vi "2016RefLoopPulseGen_Original.vi"() -> ()   [LabVIEW 2015]
uses:
  <vilib>/express/express arith-compare/Formula/XNode/ExpressFormulaBlockNode.xnode
  <vilib>/express/express shared/transition.llb/Dynamic To Waveform Array.vi
  <vilib>/express/express arith-compare/Formula/Block/exnFormulaBlock how many pts in the wave.vi
  <vilib>/express/express shared/ex_Modify Signal Name.vi
  <vilib>/express/express shared/transition.llb/Waveform Array To Dynamic.vi
  <vilib>/addons/control/pid/NI_PID_autopid.lvlib
  <vilib>/DAQmx/write.llb/DAQmx Write (Digital 1D Bool 1Chan 1Samp).vi
  <vilib>/Utility/error.llb/DialogType.ctl
  <vilib>/express/express signal manip/GetorSetDDTAttributes/Set DDT Attributes/Set DDT Properties.xnode
  <vilib>/express/express signal manip/GetorSetDDTAttributes/Set DDT Attributes/SetT0.vi
  <vilib>/DAQmx/configure/timing.llb/DAQmx Timing (Sample Clock).vi
  <vilib>/DAQmx/configure/timing.llb/DAQmx Timing (Implicit).vi
  <vilib>/DAQmx/create/channels.llb/DAQmx Create Channel (CO-Pulse Generation-Frequency).vi
  <vilib>/DAQmx/write.llb/DAQmx Write (Digital 1D Bool NChan 1Samp 1Line).vi
  <vilib>/DAQmx/read.llb/DAQmx Read (Analog 1D DBL NChan 1Samp).vi
panel:
  out "Loop Time":dbl
  in  "stop 4":bool
  in  "?":bool
  out "error out 2":errorcluster
  out "error out":errorcluster
  in  "output duty cycle range 1":cluster{"output high":dbl, "output low":dbl}={"output high"=100.0, "output low"=0.0}
  out "Waveform Chart":dbl(graph)=1.0280585289001465
  out "Elapsed Time (s)":dbl=1192.0481810569763
  in  "?":T1(tab)
  in  "Lower Test Section offset":dbl
  in  "Separator T offset":dbl
  in  "Liquid Tank P offset":dbl=8500.0
  out "Test Section P (Pa)":dbl=116198.57530062649
  in  "P atm":dbl=101325.0
  in  "Liquid Inlet Offset":dbl=1100.0
  in  "Upper Test Sec":dbl
  in  "Dev Section P offset":dbl=-15000.0
  in  "Liquid Inlet T offset":dbl
  in  "Vapor Inlet T offset":dbl
  in  "Liquid Tank T offset":dbl
  in  "Vapor Tank T offset":dbl
  in  "Separator P Offset":dbl=2500.0
  out "Liquid Tank Heater Temp. [C]":dbl=-0.00013997779130803294 format="%#_4g"
  out "Vapor Tank Heater Temp. [C]":dbl=-0.00010921620483495026 format="%#_4g"
  in  "Vapor Tank Heater [V]":dbl(slide) scale=0.0..10.0
  in  "Liquid Tank Heater [V]":dbl(slide) scale=0.0..10.0
  out "Quality\n[-]":dbl=0.5124735258578829 format="%#_3f"
  out "Mixture Enthalpy":dbl=315341.8738601937
  out "Upper TS Sat. Temp. [C]":dbl=-30.741985921320232 format="%#_4g"
  out "Upper Test Section 2\n(not connected)":dbl=19080.10707676887
  out "?":dbl=nan format="%#_4g"
  out "?":dbl=nan format="%#_4g"
  out "Vapor Inlet Sat. Temp. [C]":dbl=18.983650599672455 format="%#_4g"
  out "Liquid Inlet Sat. Temp. [C]":dbl=18.967113726868046 format="%#_4g"
  out "Separator Sat. Temp. [C]":dbl=18.962084458713754 format="%#_4g"
  out "Liquid Tank Sat. Temp. [C]":dbl=17.336038014955804 format="%#_4g"
  out "Vapor Tank Sat. Temp. [C]":dbl=nan format="%#_4g"
  out "Lower Test Section 2\n(not connected)":dbl=-5.945274707393333 format="%#_6f"
  out "Streamwise":dbl=-4309.180034596612 format="%#_2e"
  out "Dev Section":dbl=117529.39865406745 format="%#_5f"
  out "Separator 2":dbl=117436.76445279745 format="%#_5f"
  out "Vapor Tank 2\n(need replaced)":dbl=-34009.73110511369 format="%#_6f"
  out "Liquid Inlet 2":dbl=117458.36040777806 format="%#_5f"
  out "Liquid Tank 2":dbl=119158.55398835387 format="%#_5f"
  out "Upper TS Sat. Pres.":dbl=117745.79282373996
  out "Upper Test Section":dbl=19.02953821278611 format="%#_4g"
  out "Lower Test Section":dbl=18.841711969674257 format="%#_4g"
  out "Vapor Inlet":dbl=19.940090617924646 format="%#_4g"
  out "Liquid Inlet":dbl=19.29273815741822 format="%#_4g"
  out "Separator":dbl=19.351746784304748 format="%#_4g"
  out "Liquid Tank":dbl=19.064732737324512 format="%#_4g"
  out "Vapor Tank":dbl=19.311251471245498 format="%#_4g"
  out "Liquid Inlet Sat. Pres.":dbl=118921.18754866866 format="%#_4f"
  out "Liquid Tank Sat. Pres.":dbl=117902.28866165497 format="%#_4f"
  out "Vapor Inlet Sat. Pres.":dbl=119186.31350697557 format="%#_4f"
  out "Lower Test Section Sat. Pres.":dbl=116914.11104502712 format="%#_4f"
  out "Separator Sat. Pres.":dbl=121862.28710047182 format="%#_4f"
  out "Vapor Tank Sat. Pres.":dbl=119004.3043776936 format="%#_4f"
  out "Evaporator Bottom":dbl=0.07812510710210246 format="%#_4g"
  out "Evaporator Top":dbl=-55440.10937765434 format="%#_4g"
  out "Condenser Bottom":dbl=-0.00013633631982423782 format="%#_4g"
  out "Condenser Top":dbl=-0.0001304783004807413 format="%#_4g"
  in  "Save File":bool
  out "StaticPressDiff(Pa)":dbl=-222.00009683752145
  out "DC":dbl
  out "Numeric":dbl=2.098083621149279e-08
  out "Pressure Drop":dbl=2.6226045264365988e-08
  in  "Boolean 2":bool
  out "Camera Voltage":dynamicdata(graph)
  in  "Pitot Offset [Pa]":dbl
  in  "PG-TS Offset\n[Pa]":dbl
  in  "Send Pulse 2":bool
  out "Psat liq":dbl=119.96937909943745
  in  "Save Loop Data":bool
  in  "Boolean":bool
  in  "Sampling frequency (Hz)":dbl=1000.0
  in  "Length of recording (s)":dbl=2.0
  in  "PG Abs Offset":dbl=11500.0
  out "Psat vap":dbl=121.24568157832624
  out "Pitot Amps":dbl=2.6415199999999147e-07
  out "dP Pitot Probe":dynamicdata(graph)=[{"t0"=timestamp(3554308544.5452676 s since 1904-01-01), "dt"=0.001, "Y"=array[2000 elements], "attributes"=variant("NI_ChannelName"=variant(string "Pitot dP (Formula Result)"), "NI_OriginalChannelName"=variant(string "Pitot dP"), "NI_UnitDescription"=variant(string "Amps"))}]
  out "Tank Pressure":dynamicdata(graph)=[{"t0"=timestamp(3554308544.5452676 s since 1904-01-01), "dt"=0.001, "Y"=array[2000 elements], "attributes"=variant("NI_ChannelName"=variant(string "Abs P (Formula Result)"), "NI_OriginalChannelName"=variant(string "Abs P"), "NI_UnitDescription"=variant(string "Volts"))}]
  out "dP to test section":dynamicdata(graph)=[{"t0"=timestamp(3554308544.5452814 s since 1904-01-01), "dt"=0.001, "Y"=array[2000 elements], "attributes"=variant("NI_ChannelName"=variant(string "PG to TS dP (Formula Result)"), "NI_OriginalChannelName"=variant(string "PG to TS dP"), "NI_UnitDescription"=variant(string "Volts"))}]
  out "Pitot dP":dbl=-4308.9404273994505
  out "Liquid Temp":dbl=19.52526901660894
  out "Vapor Temp":dbl=19.805676371442082
  in  "CCW":bool
  in  "?":bool
  out "Loop iterations":i32
  in  "Send Pulse":bool
  in  "Steps":i32=10000 min=0 max=40000 step=500
  in  "Idle State":i32(ring)=10214 items=["High"=10192, "Low"=10214]
  in  "Counter(s)":tag="cDAQ1Mod8/ctr0" caption="Counter"
  in  "Duty Cycle":dbl=0.5 min=0.1 max=1.0 step=0.1
  in  "Frequency (Hz)":dbl=1000.0 min=0.0 max=10000.0 step=500.0
  out "Mass Flow Rate":dbl=nan
  in  "Heaters":bool
  out "PG Abs":dbl=119484.80284900061
  out "PG to TS dP":dbl=4351.8068090218785
  in  "Save dP data":bool
  out "dP [Pa]  W1 to W7":dbl=-0.008208439355650089
  out "dP [Pa] W1 to W4":dbl=0.008075495341450085
  in  "stop":bool
  in  "reinitialize? (F) 2":bool=TRUE
  out "Liquid Mass Flow Rate":cluster{"[0]":dbl, "[1]":dbl}(graph)={"[0]"=0.0, "[1]"=-94.2977673785965}
  out "Voltage Out 2":dbl
  out "Liquid Line Density [g/cm3]":dbl=-0.5000013113022632
  out "Liquid Flow Rate [g/s]":dbl=-94.2977673785965
  in  "LiquidOnOff":bool
  in  "LiquidManPID":bool
  in  "PID gains 2":T2={"proportional gain (Kc)"=1e-15, "integral time (Ti, min)"=1e-12, "derivative time (Td, min)"=1e-12} {"derivative time (Td, min)" format="%.4e"; "integral time (Ti, min)" format="%.4e"; "proportional gain (Kc)" format="%.4e"}
  in  "output range 2":cluster{"output high":dbl, "output low":dbl}={"output high"=4.5, "output low"=2.0} {"output low" format="%.2f"; "output high" format="%.2f"}
  in  "Valve Voltage [V] 2":dbl=2.6 format="%.2f"
  in  "Liquid Flow Set Point\n[g/s]":dbl format="%.2f"
  in  "output range":cluster{"output high":dbl, "output low":dbl}={"output high"=3.0, "output low"=2.0} {"output low" format="%.2f"; "output high" format="%.2f"}
  in  "PID gains":T2={"proportional gain (Kc)"=1e-14, "integral time (Ti, min)"=1e-12, "derivative time (Td, min)"=1e-12} {"derivative time (Td, min)" format="%.4e"; "integral time (Ti, min)" format="%.4e"; "proportional gain (Kc)" format="%.4e"}
  in  "VaporManPID":bool
  in  "VaporOnOff":bool
  in  "Vapor Flow Set Point\n[g/s]":dbl format="%.2f"
  in  "Valve Voltage [V]":dbl=2.33 format="%.2f"
  out "Vapor Line Density [g/cm3]":dbl=-0.5000029504300922
  out "Vapor Flow Rate [g/s]":dbl=-94.29782933653023
  out "Voltage Out":dbl
  out "Vapor Mass Flow Rate":cluster{"[0]":dbl, "[1]":dbl}(graph)
  in  "reinitialize? (F)":bool=TRUE
  in  "PID on 2":bool
  in  "T1 Setpoint [C]":dbl format="%.2f"
  in  "reinitialize? (F) 3":bool=TRUE
  in  "PID gains 3":T2={"proportional gain (Kc)"=1e-14, "integral time (Ti, min)"=1e-12, "derivative time (Td, min)"=1e-12} {"derivative time (Td, min)" format="%.4e"; "integral time (Ti, min)" format="%.4e"; "proportional gain (Kc)" format="%.4e"}
  out "T1":cluster{"[0]":dbl, "[1]":dbl}(graph)
  out "T1 Measured [C]":dbl
  out "DutyCycleCalc1":dbl format="%.6f"
  in  "T2 Setpoint [C]":dbl format="%.2f"
  in  "reinitialize? (F) 4":bool=TRUE
  in  "PID gains 4":T2={"proportional gain (Kc)"=1e-14, "integral time (Ti, min)"=1e-12, "derivative time (Td, min)"=1e-12} {"derivative time (Td, min)" format="%.4e"; "integral time (Ti, min)" format="%.4e"; "proportional gain (Kc)" format="%.4e"}
  out "T2":cluster{"[0]":dbl, "[1]":dbl}(graph)
  out "T2 Measured [C]":dbl
  out "DutyCycleCalc2":dbl format="%.6f"
  in  "stop 2":bool
  in  "PID on":bool
  in  "PID on 3":bool
  in  "T3 Setpoint [C]":dbl format="%.2f"
  in  "reinitialize? (F) 5":bool=TRUE
  in  "PID gains 5":T2={"proportional gain (Kc)"=1e-14, "integral time (Ti, min)"=1e-12, "derivative time (Td, min)"=1e-12} {"derivative time (Td, min)" format="%.4e"; "integral time (Ti, min)" format="%.4e"; "proportional gain (Kc)" format="%.4e"}
  out "T3":cluster{"[0]":dbl, "[1]":dbl}(graph)
  out "T3 Measured [C]":dbl
  out "DutyCycleCalc3":dbl format="%.6f"
  in  "PID on 4":bool
  in  "T4 Setpoint [C]":dbl format="%.2f"
  in  "reinitialize? (F) 6":bool=TRUE
  in  "PID gains 6":T2={"proportional gain (Kc)"=1e-14, "integral time (Ti, min)"=1e-12, "derivative time (Td, min)"=1e-12} {"derivative time (Td, min)" format="%.4e"; "integral time (Ti, min)" format="%.4e"; "proportional gain (Kc)" format="%.4e"}
  out "T4":cluster{"[0]":dbl, "[1]":dbl}(graph)
  out "T4 Measured [C]":dbl
  out "DutyCycleCalc4":dbl format="%.6f"
  in  "PID on 5":bool
  in  "T5 Setpoint [C]":dbl format="%.2f"
  in  "reinitialize? (F) 7":bool=TRUE
  in  "PID gains 7":T2={"proportional gain (Kc)"=1e-14, "integral time (Ti, min)"=1e-12, "derivative time (Td, min)"=1e-12} {"derivative time (Td, min)" format="%.4e"; "integral time (Ti, min)" format="%.4e"; "proportional gain (Kc)" format="%.4e"}
  out "T5":cluster{"[0]":dbl, "[1]":dbl}(graph)
  out "T5 Measured [C]":dbl
  out "DutyCycleCalc5":dbl format="%.6f"
  in  "PID on 6":bool
  in  "T6 Setpoint [C]":dbl format="%.2f"
  in  "reinitialize? (F) 8":bool=TRUE
  in  "PID gains 8":T2={"proportional gain (Kc)"=1e-14, "integral time (Ti, min)"=1e-12, "derivative time (Td, min)"=1e-12} {"derivative time (Td, min)" format="%.4e"; "integral time (Ti, min)" format="%.4e"; "proportional gain (Kc)" format="%.4e"}
  out "T6":cluster{"[0]":dbl, "[1]":dbl}(graph)
  out "T6 Measured [C]":dbl
  out "DutyCycleCalc6":dbl format="%.6f"
  in  "PID on 7":bool
  in  "T7 Setpoint [C]":dbl format="%.2f"
  in  "reinitialize? (F) 9":bool=TRUE
  in  "PID gains 9":T2={"proportional gain (Kc)"=1e-14, "integral time (Ti, min)"=1e-12, "derivative time (Td, min)"=1e-12} {"derivative time (Td, min)" format="%.4e"; "integral time (Ti, min)" format="%.4e"; "proportional gain (Kc)" format="%.4e"}
  out "T7":cluster{"[0]":dbl, "[1]":dbl}(graph)
  out "T7 Measured [C]":dbl
  out "DutyCycleCalc7":dbl format="%.6f"
  out "WinOn 2":bool
  out "WinOn 1":bool
  in  "PID on 8":bool
  in  "T8 Setpoint [C]":dbl format="%.2f"
  in  "reinitialize? (F) 10":bool=TRUE
  in  "PID gains 10":T2={"proportional gain (Kc)"=1e-14, "integral time (Ti, min)"=1e-12, "derivative time (Td, min)"=1e-12} {"derivative time (Td, min)" format="%.4e"; "integral time (Ti, min)" format="%.4e"; "proportional gain (Kc)" format="%.4e"}
  out "T8":cluster{"[0]":dbl, "[1]":dbl}(graph)
  out "T8 Measured [C]":dbl
  out "DutyCycleCalc8":dbl format="%.6f"
  in  "PID on 9":bool
  in  "T9 Setpoint [C]":dbl format="%.2f"
  in  "reinitialize? (F) 11":bool=TRUE
  in  "PID gains 11":T2={"proportional gain (Kc)"=1e-14, "integral time (Ti, min)"=1e-12, "derivative time (Td, min)"=1e-12} {"derivative time (Td, min)" format="%.4e"; "integral time (Ti, min)" format="%.4e"; "proportional gain (Kc)" format="%.4e"}
  out "T9":cluster{"[0]":dbl, "[1]":dbl}(graph)
  out "T9 Measured [C]":dbl
  out "DutyCycleCalc9":dbl format="%.6f"
  in  "PID on 10":bool
  in  "T10 Setpoint [C]":dbl format="%.2f"
  in  "reinitialize? (F) 12":bool=TRUE
  in  "PID gains 12":T2={"proportional gain (Kc)"=1e-14, "integral time (Ti, min)"=1e-12, "derivative time (Td, min)"=1e-12} {"derivative time (Td, min)" format="%.4e"; "integral time (Ti, min)" format="%.4e"; "proportional gain (Kc)" format="%.4e"}
  out "T10":cluster{"[0]":dbl, "[1]":dbl}(graph)
  out "T10 Measured [C]":dbl
  out "DutyCycleCalc10":dbl format="%.6f"
  in  "PID on 11":bool
  in  "T11 Setpoint [C]":dbl format="%.2f"
  in  "reinitialize? (F) 13":bool=TRUE
  in  "PID gains 13":T2={"proportional gain (Kc)"=1e-14, "integral time (Ti, min)"=1e-12, "derivative time (Td, min)"=1e-12} {"derivative time (Td, min)" format="%.4e"; "integral time (Ti, min)" format="%.4e"; "proportional gain (Kc)" format="%.4e"}
  out "T11":cluster{"[0]":dbl, "[1]":dbl}(graph)
  out "T11 Measured [C]":dbl
  out "DutyCycleCalc11":dbl format="%.6f"
  in  "PID on 12":bool
  in  "T12 Setpoint [C]":dbl format="%.2f"
  in  "reinitialize? (F) 14":bool=TRUE
  in  "PID gains 14":T2={"proportional gain (Kc)"=1e-14, "integral time (Ti, min)"=1e-12, "derivative time (Td, min)"=1e-12} {"derivative time (Td, min)" format="%.4e"; "integral time (Ti, min)" format="%.4e"; "proportional gain (Kc)" format="%.4e"}
  out "T12":cluster{"[0]":dbl, "[1]":dbl}(graph)
  out "T12 Measured [C]":dbl
  out "DutyCycleCalc12":dbl format="%.6f"
  in  "PID on 13":bool
  in  "T13 Setpoint [C]":dbl format="%.2f"
  in  "reinitialize? (F) 15":bool=TRUE
  in  "PID gains 15":T2={"proportional gain (Kc)"=1e-14, "integral time (Ti, min)"=1e-12, "derivative time (Td, min)"=1e-12} {"derivative time (Td, min)" format="%.4e"; "integral time (Ti, min)" format="%.4e"; "proportional gain (Kc)" format="%.4e"}
  out "T13":cluster{"[0]":dbl, "[1]":dbl}(graph)
  out "T13 Measured [C]":dbl
  out "DutyCycleCalc13":dbl format="%.6f"
  in  "PID on 14":bool
  in  "T14 Setpoint [C]":dbl format="%.2f"
  in  "reinitialize? (F) 16":bool=TRUE
  in  "PID gains 16":T2={"proportional gain (Kc)"=1e-14, "integral time (Ti, min)"=1e-12, "derivative time (Td, min)"=1e-12} {"derivative time (Td, min)" format="%.4e"; "integral time (Ti, min)" format="%.4e"; "proportional gain (Kc)" format="%.4e"}
  out "T14":cluster{"[0]":dbl, "[1]":dbl}(graph)
  out "T14 Measured [C]":dbl
  out "DutyCycleCalc14":dbl format="%.6f"
  # "Same button as Save data loop button on Pulse Generator tab"
  # "Test Section Properties"
  # "Pressure\n[Pa]"
  # "Sat. Temp.\n[C]"
  # "Sat. Pressure\n[Pa]"
  # "Temp.\n[C]"
  # "Temperature [C]"
  # "Condenser"
  # "Evaporator"
  # "Top"
  # "Bottom"
  # "Save File"
  # "Do Not\nSave File"
  # "In order to send a  group of pulses follow the steps below.\n1)Press the button labeled Send Pulse\n2)Press the button a second time in order to prepare for another pulse\n3)Press the stop button to reset the Send Pulse button\n4)Repeat process for next pulse\n\nNote: 1000 steps is a full cycle of the valve, this will send one pulse"
  # "Saving Data:\n\n- Press the Save Loop Data button to record time-averaged (every 2s) data from the loop (data from Test Section Properties tab). Pressing the button again keeps writing in the same file.\n\n-Press the Save dP data to record time resolved data. Each time you press the button, a new file is recorded."
  # "Pulse Generator\nTemperatures"
  # "Vapor Side"
  # "Valve On"
  # "Valve Off"
  # "Manual Flow\nControl"
  # "PID Flow\nControl"
  # "Liquid Side"
  # "Valve On"
  # "Valve Off"
  # "Manual Flow\nControl"
  # "PID Flow\nControl"
  # "Heater On"
  # "Heater On"
  # "Heater On"
  # "Heater On"
  # "Heater Off"
  # "Heater Off"
  # "Heater Off"
  # "Heater Off"
  # "Heater On"
  # "Heater On"
  # "Heater On"
  # "Heater Off"
  # "Heater Off"
  # "Heater Off"
  # "Heater On"
  # "Heater On"
  # "Heater On"
  # "Heater On"
  # "Heater Off"
  # "Heater Off"
  # "Heater Off"
  # "Heater Off"
  # "Heater On"
  # "Heater On"
  # "Heater On"
  # "Heater Off"
  # "Heater Off"
  # "Heater Off"
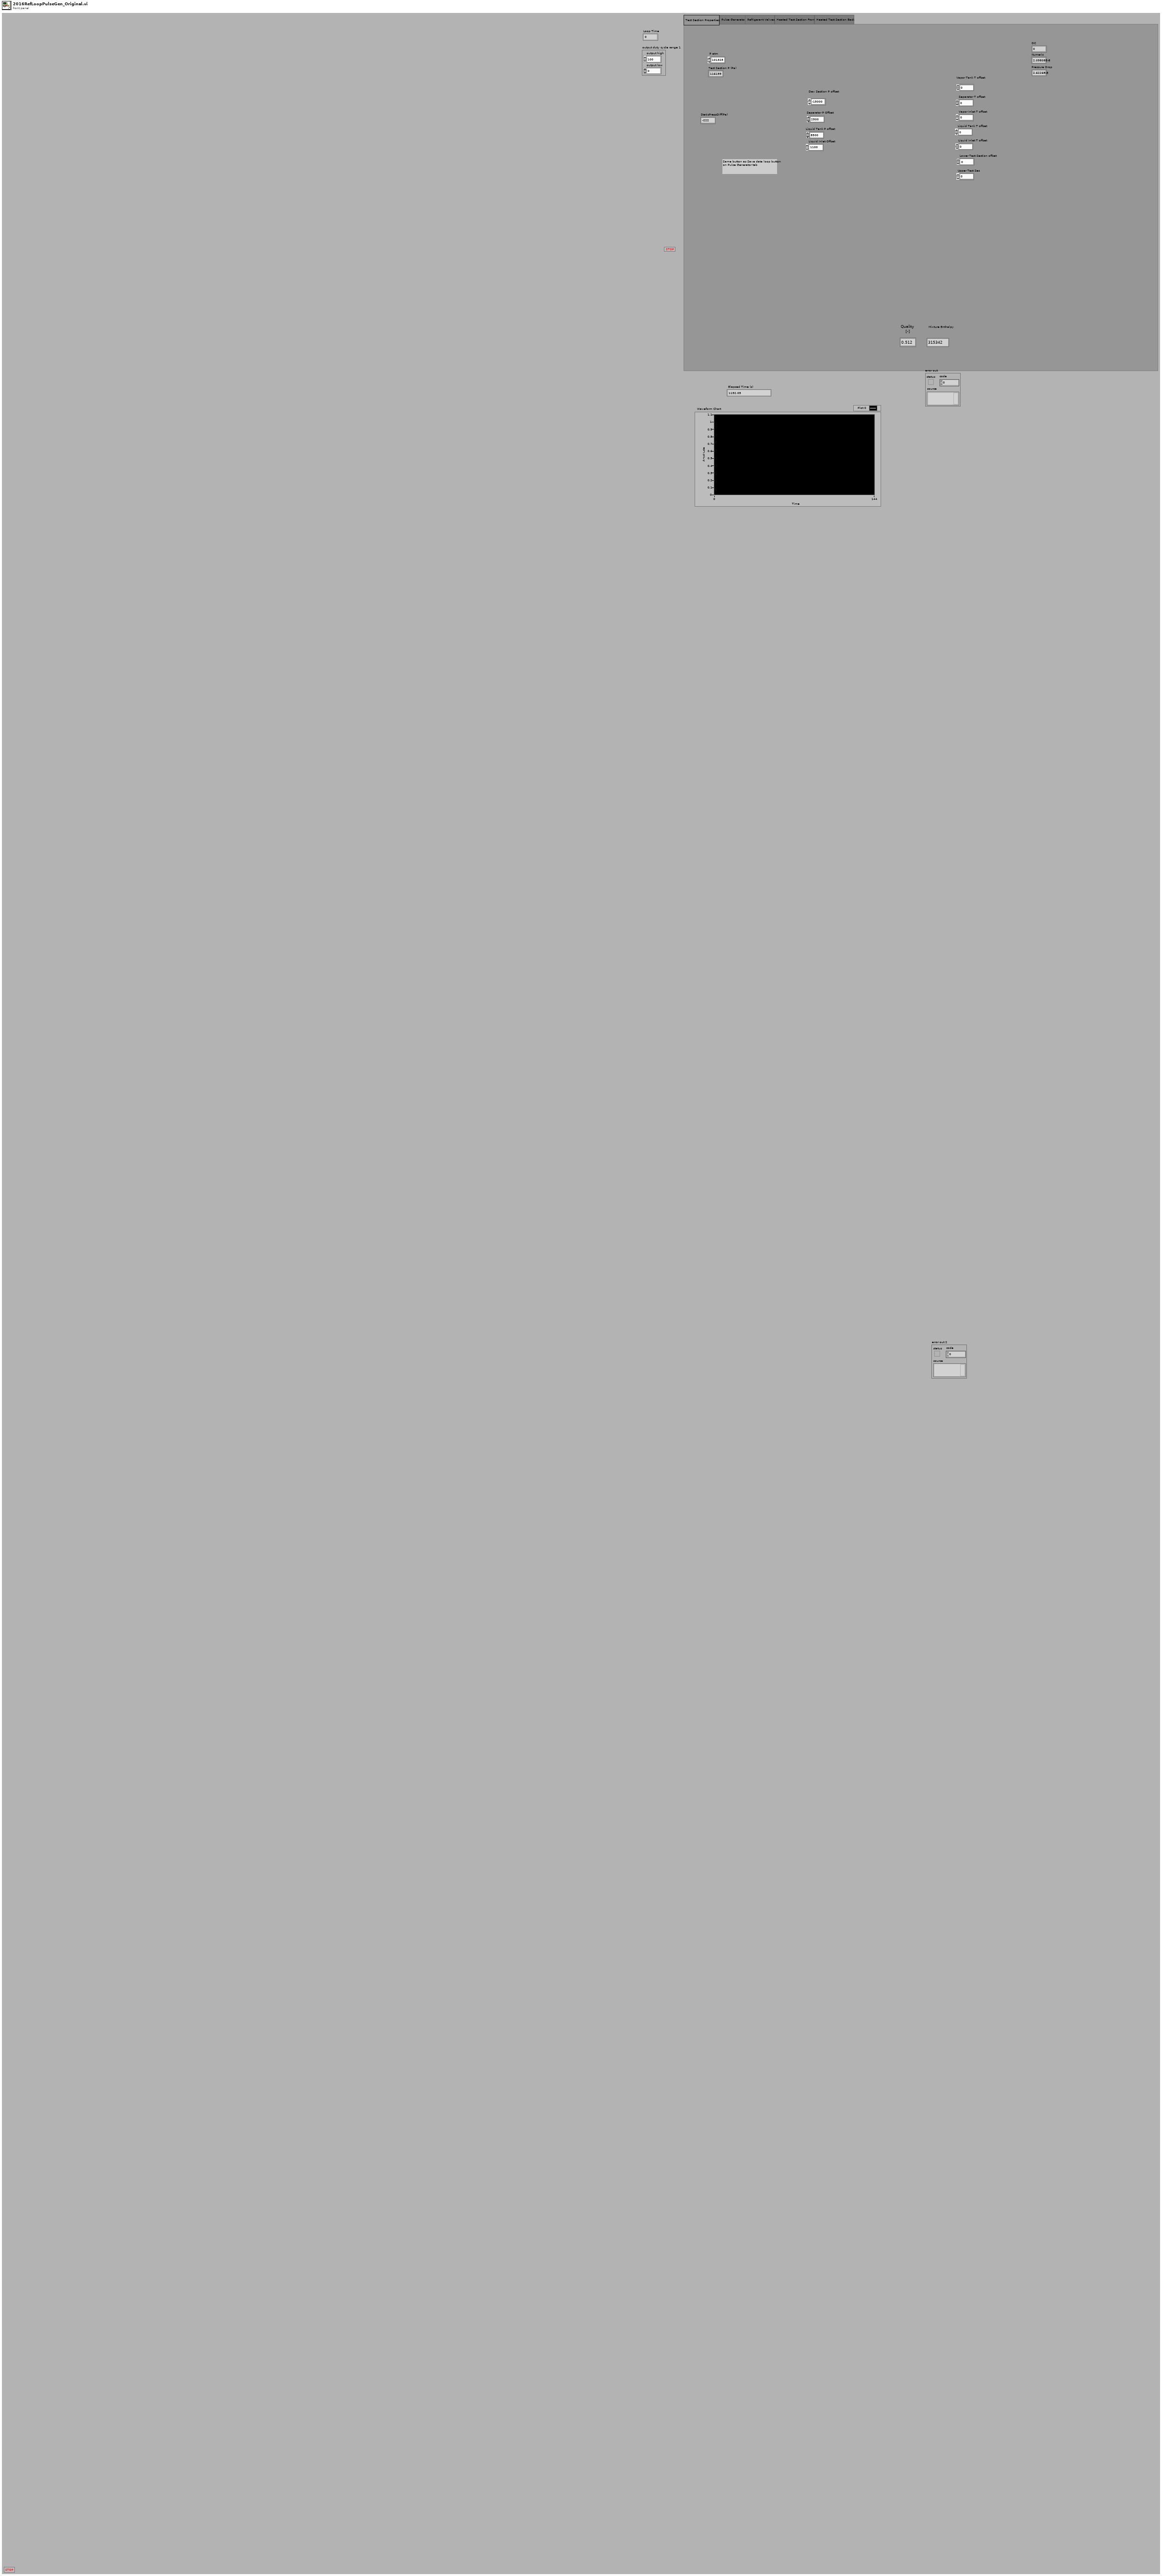
[diagram p1: front panel]
types:
  T1 = enum32{"Test Section Properties", "Pulse Generator", "Refrigerant Valves", "Heated Test Section Front", "Heated Test Section Back"}
  T2 = cluster{"proportional gain (Kc)":dbl, "integral time (Ti, min)":dbl, "derivative time (Td, min)":dbl}
  T3 = typedef "DialogType.ctl" = u16
  T4 = cluster{bool[], bool[], bool[], bool[], bool[], bool[], bool[], bool[], bool[], bool[], bool[], bool[], bool[], bool[]}
  T5 = cluster{"controller type":u16, "relay cycles":i32, "relay amplitude":dbl, "control specification":u16, "PV noise level":dbl}
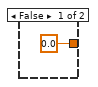
[diagram p6: hidden frame]
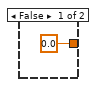
[diagram p7: hidden frame]
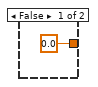
[diagram p8: hidden frame]
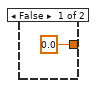
[diagram p9: hidden frame]
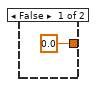
[diagram p10: hidden frame]
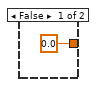
[diagram p11: hidden frame]
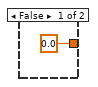
[diagram p12: hidden frame]
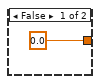
[diagram p13: hidden frame]
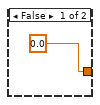
[diagram p14: hidden frame]
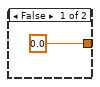
[diagram p15: hidden frame]
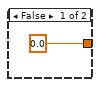
[diagram p16: hidden frame]
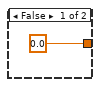
[diagram p17: hidden frame]
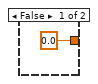
[diagram p18: hidden frame]
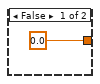
[diagram p19: hidden frame]
diagram:
  w1 = T3 3 items=["no dialog", "OK message", "continue or stop message", "OK message + warnings", "continue/stop + warnings"] ("type of dialog (OK msg:1)")
  w11 = refnum<k21> "DigitalTaskOut1"  # DAQmx Task Name
  w19 = refnum<k21> "HeatedTSWindows"  # DAQmx Task Name
  n1 = call <vilib>:"DAQmx Start Task.vi"("task/channels in"=w19) -> ("task out"=w18:refnum<k21>, "error out"=w17:errorcluster)  [unwired: 13 in]
  n2 = call <vilib>:"DAQmx Start Task.vi"("task/channels in"=w11) -> ("task out"=w10:refnum<k21>, "error out"=w9:errorcluster)  [unwired: 13 in]
  n3 = while {
    shift-right: [w171] -> _
    shift-left: 0.0 ("Elapsed Time (s)") -> [w170]
    tunnel: w18 -> [w54]
    tunnel: w17 -> [w53]
    tunnel: [w52] -> w16
    tunnel: [w51] -> w15
    tunnel: w10 -> [w31]
    tunnel: w9 -> [w30]
    tunnel: [w29] -> w6
    tunnel: [w28] -> w5
    shift-right: [w34] -> _
    shift-left: T4 {[FALSE], [FALSE], [], [], [], [], [], [], [], [], [], [], [], []} -> [w49]
    stop <- "stop 2" stop-if-true
    w32 = i64 100 ("Length 2")
    w95 = T5 {"controller type"=1, "relay cycles"=3, "relay amplitude"=1.0, "control specification"=2, "PV noise level"=0.1} ("autotuning parameters")
    # "Replace with Measured Temp"
    # "Replace with Measured Temp"
    n4 = call-poly <vilib>:"DAQmx Read.vi"("task/channels in"=w54, "error in"=w53) -> ("task out"=w52:refnum<k21>, "data"=w50:dbl[], "error out"=w51:errorcluster)  [unwired: 11 in]
    n5 = Index Array(array=w50, index #1=1 ("index"), index #2=2 ("index"), index #3=3 ("index"), index #4=4 ("index"), index #5=5 ("index"), index #6=6 ("index"), index #7=7 ("index"), index #8=8 ("index"), index #9=9 ("index"), index #10=10 ("index"), index #11=11 ("index"), index #12=12 ("index"), index #13=13 ("index"), index #14=14 ("index")) -> (element #1=w68:dbl, element #2=w67:dbl, element #3=w66:dbl, element #4=w65:dbl, element #5=w64:dbl, element #6=w63:dbl, element #7=w62:dbl, element #8=w61:dbl, element #9=w60:dbl, element #10=w59:dbl, element #11=w58:dbl, element #12=w57:dbl, element #13=w56:dbl, element #14=w55:dbl)
    "T1 Measured [C]" <- w68
    "T2 Measured [C]" <- w67
    "T3 Measured [C]" <- w66
    "T4 Measured [C]" <- w65
    "T5 Measured [C]" <- w64
    "T6 Measured [C]" <- w63
    "T7 Measured [C]" <- w62
    "T8 Measured [C]" <- w61
    "T9 Measured [C]" <- w60
    "T10 Measured [C]" <- w59
    "T11 Measured [C]" <- w58
    "T12 Measured [C]" <- w57
    "T13 Measured [C]" <- w56
    "T14 Measured [C]" <- w55
    n6 = Build Array("T1 Setpoint [C]", w68) -> (w168:dbl[])
    n7 = Build Array("T2 Setpoint [C]", w67) -> (w161:dbl[])
    n8 = Build Array("T3 Setpoint [C]", w66) -> (w155:dbl[])
    n9 = Build Array("T4 Setpoint [C]", w65) -> (w150:dbl[])
    n10 = Array To Cluster(array=w168) -> (cluster=→"T1":cluster{"[0]":dbl, "[1]":dbl})
    n11 = Array To Cluster(array=w161) -> (cluster=→"T2":cluster{"[0]":dbl, "[1]":dbl})
    n12 = Array To Cluster(array=w155) -> (cluster=→"T3":cluster{"[0]":dbl, "[1]":dbl})
    n13 = Array To Cluster(array=w150) -> (cluster=→"T4":cluster{"[0]":dbl, "[1]":dbl})
    n14 = case shown="True" "PID on" {
      tunnel: "T1 Setpoint [C]" -> [_ w340]
      tunnel: [0.0 ("output") w337] -> w164
      tunnel: w68 -> [_ w339]
      tunnel: "output duty cycle range 1" -> [_ w336]
      tunnel: w95 -> [_ w335]
      frame False {
      }
      frame True {
        n15 = call <vilib>:"PID Autotuning.vi"("autotuning parameters"=w335, "reinitialize? (F)"="reinitialize? (F) 3", "output range"=w336, "PID gains"="PID gains 3", "process variable"=w339, "setpoint"=w340) -> ("output"=w337:dbl)  [unwired: 2 in, 3 out]
      }
    }
    "DutyCycleCalc1" <- w164
    n16 = case shown="True" "PID on 6" {
      tunnel: "T6 Setpoint [C]" -> [_ w300]
      tunnel: [0.0 ("output") w297] -> w137
      tunnel: w63 -> [_ w299]
      tunnel: "output duty cycle range 1" -> [_ w296]
      tunnel: w95 -> [_ w295]
      frame False {
      }
      frame True {
        n17 = call <vilib>:"PID Autotuning.vi"("autotuning parameters"=w295, "reinitialize? (F)"="reinitialize? (F) 8", "output range"=w296, "PID gains"="PID gains 8", "process variable"=w299, "setpoint"=w300) -> ("output"=w297:dbl)  [unwired: 2 in, 3 out]
      }
    }
    "DutyCycleCalc6" <- w137
    n18 = case shown="True" "PID on 3" {
      tunnel: "T3 Setpoint [C]" -> [_ w324]
      tunnel: [0.0 ("output") w321] -> w152
      tunnel: w66 -> [_ w323]
      tunnel: "output duty cycle range 1" -> [_ w320]
      tunnel: w95 -> [_ w319]
      frame False {
      }
      frame True {
        n19 = call <vilib>:"PID Autotuning.vi"("autotuning parameters"=w319, "reinitialize? (F)"="reinitialize? (F) 5", "output range"=w320, "PID gains"="PID gains 5", "process variable"=w323, "setpoint"=w324) -> ("output"=w321:dbl)  [unwired: 2 in, 3 out]
      }
    }
    "DutyCycleCalc3" <- w152
    n20 = case shown="True" "PID on 12" {
      tunnel: "T12 Setpoint [C]" -> [_ w252]
      tunnel: [0.0 ("output") w249] -> w107
      tunnel: w57 -> [_ w251]
      tunnel: "output duty cycle range 1" -> [_ w248]
      tunnel: w95 -> [_ w247]
      frame False {
      }
      frame True {
        n21 = call <vilib>:"PID Autotuning.vi"("autotuning parameters"=w247, "reinitialize? (F)"="reinitialize? (F) 14", "output range"=w248, "PID gains"="PID gains 14", "process variable"=w251, "setpoint"=w252) -> ("output"=w249:dbl)  [unwired: 2 in, 3 out]
      }
    }
    "DutyCycleCalc12" <- w107
    n22 = case shown="True" "PID on 13" {
      tunnel: "T13 Setpoint [C]" -> [_ w244]
      tunnel: [0.0 ("output") w241] -> w102
      tunnel: w56 -> [_ w243]
      tunnel: "output duty cycle range 1" -> [_ w240]
      tunnel: w95 -> [_ w239]
      frame False {
      }
      frame True {
        n23 = call <vilib>:"PID Autotuning.vi"("autotuning parameters"=w239, "reinitialize? (F)"="reinitialize? (F) 15", "output range"=w240, "PID gains"="PID gains 15", "process variable"=w243, "setpoint"=w244) -> ("output"=w241:dbl)  [unwired: 2 in, 3 out]
      }
    }
    "DutyCycleCalc13" <- w102
    n24 = case shown="True" "PID on 10" {
      tunnel: "T10 Setpoint [C]" -> [_ w268]
      tunnel: [0.0 ("output") w265] -> w117
      tunnel: w59 -> [_ w267]
      tunnel: "output duty cycle range 1" -> [_ w264]
      tunnel: w95 -> [_ w263]
      frame False {
      }
      frame True {
        n25 = call <vilib>:"PID Autotuning.vi"("autotuning parameters"=w263, "reinitialize? (F)"="reinitialize? (F) 12", "output range"=w264, "PID gains"="PID gains 12", "process variable"=w267, "setpoint"=w268) -> ("output"=w265:dbl)  [unwired: 2 in, 3 out]
      }
    }
    "DutyCycleCalc10" <- w117
    n26 = case shown="True" "PID on 2" {
      tunnel: "T2 Setpoint [C]" -> [_ w332]
      tunnel: [0.0 ("output") w329] -> w158
      tunnel: w67 -> [_ w331]
      tunnel: "output duty cycle range 1" -> [_ w328]
      tunnel: w95 -> [_ w327]
      frame False {
      }
      frame True {
        n27 = call <vilib>:"PID Autotuning.vi"("autotuning parameters"=w327, "reinitialize? (F)"="reinitialize? (F) 4", "output range"=w328, "PID gains"="PID gains 4", "process variable"=w331, "setpoint"=w332) -> ("output"=w329:dbl)  [unwired: 2 in, 3 out]
      }
    }
    "DutyCycleCalc2" <- w158
    n28 = case shown="True" "PID on 9" {
      tunnel: "T9 Setpoint [C]" -> [_ w276]
      tunnel: [0.0 ("output") w273] -> w122
      tunnel: w60 -> [_ w275]
      tunnel: "output duty cycle range 1" -> [_ w272]
      tunnel: w95 -> [_ w271]
      frame False {
      }
      frame True {
        n29 = call <vilib>:"PID Autotuning.vi"("autotuning parameters"=w271, "reinitialize? (F)"="reinitialize? (F) 11", "output range"=w272, "PID gains"="PID gains 11", "process variable"=w275, "setpoint"=w276) -> ("output"=w273:dbl)  [unwired: 2 in, 3 out]
      }
    }
    "DutyCycleCalc9" <- w122
    n30 = case shown="True" "PID on 4" {
      tunnel: "T4 Setpoint [C]" -> [_ w316]
      tunnel: [0.0 ("output") w313] -> w147
      tunnel: w65 -> [_ w315]
      tunnel: "output duty cycle range 1" -> [_ w312]
      tunnel: w95 -> [_ w311]
      frame False {
      }
      frame True {
        n31 = call <vilib>:"PID Autotuning.vi"("autotuning parameters"=w311, "reinitialize? (F)"="reinitialize? (F) 6", "output range"=w312, "PID gains"="PID gains 6", "process variable"=w315, "setpoint"=w316) -> ("output"=w313:dbl)  [unwired: 2 in, 3 out]
      }
    }
    "DutyCycleCalc4" <- w147
    n32 = case shown="True" "PID on 11" {
      tunnel: "T11 Setpoint [C]" -> [_ w260]
      tunnel: [0.0 ("output") w257] -> w112
      tunnel: w58 -> [_ w259]
      tunnel: "output duty cycle range 1" -> [_ w256]
      tunnel: w95 -> [_ w255]
      frame False {
      }
      frame True {
        n33 = call <vilib>:"PID Autotuning.vi"("autotuning parameters"=w255, "reinitialize? (F)"="reinitialize? (F) 13", "output range"=w256, "PID gains"="PID gains 13", "process variable"=w259, "setpoint"=w260) -> ("output"=w257:dbl)  [unwired: 2 in, 3 out]
      }
    }
    "DutyCycleCalc11" <- w112
    n34 = case shown="True" "PID on 5" {
      tunnel: "T5 Setpoint [C]" -> [_ w308]
      tunnel: [0.0 ("output") w305] -> w142
      tunnel: w64 -> [_ w307]
      tunnel: "output duty cycle range 1" -> [_ w304]
      tunnel: w95 -> [_ w303]
      frame False {
      }
      frame True {
        n35 = call <vilib>:"PID Autotuning.vi"("autotuning parameters"=w303, "reinitialize? (F)"="reinitialize? (F) 7", "output range"=w304, "PID gains"="PID gains 7", "process variable"=w307, "setpoint"=w308) -> ("output"=w305:dbl)  [unwired: 2 in, 3 out]
      }
    }
    "DutyCycleCalc5" <- w142
    n36 = case shown="True" "PID on 8" {
      tunnel: "T8 Setpoint [C]" -> [_ w284]
      tunnel: [0.0 ("output") w281] -> w127
      tunnel: w61 -> [_ w283]
      tunnel: "output duty cycle range 1" -> [_ w280]
      tunnel: w95 -> [_ w279]
      frame False {
      }
      frame True {
        n37 = call <vilib>:"PID Autotuning.vi"("autotuning parameters"=w279, "reinitialize? (F)"="reinitialize? (F) 10", "output range"=w280, "PID gains"="PID gains 10", "process variable"=w283, "setpoint"=w284) -> ("output"=w281:dbl)  [unwired: 2 in, 3 out]
      }
    }
    "DutyCycleCalc8" <- w127
    n38 = case shown="True" "PID on 7" {
      tunnel: "T7 Setpoint [C]" -> [_ w292]
      tunnel: [0.0 ("output") w289] -> w132
      tunnel: w62 -> [_ w291]
      tunnel: "output duty cycle range 1" -> [_ w288]
      tunnel: w95 -> [_ w287]
      frame False {
      }
      frame True {
        n39 = call <vilib>:"PID Autotuning.vi"("autotuning parameters"=w287, "reinitialize? (F)"="reinitialize? (F) 9", "output range"=w288, "PID gains"="PID gains 9", "process variable"=w291, "setpoint"=w292) -> ("output"=w289:dbl)  [unwired: 2 in, 3 out]
      }
    }
    "DutyCycleCalc7" <- w132
    n40 = case shown="True" "PID on 14" {
      tunnel: "T14 Setpoint [C]" -> [_ w236]
      tunnel: [0.0 ("output") w233] -> w97
      tunnel: w55 -> [_ w235]
      tunnel: "output duty cycle range 1" -> [_ w232]
      tunnel: w95 -> [_ w231]
      frame False {
      }
      frame True {
        n41 = call <vilib>:"PID Autotuning.vi"("autotuning parameters"=w231, "reinitialize? (F)"="reinitialize? (F) 16", "output range"=w232, "PID gains"="PID gains 16", "process variable"=w235, "setpoint"=w236) -> ("output"=w233:dbl)  [unwired: 2 in, 3 out]
      }
    }
    "DutyCycleCalc14" <- w97
    n42 = To Quad Integer(1:w164) -> (0:w165:i64)
    n43 = To Quad Integer(1:w137) -> (0:w91:i64)
    n44 = To Quad Integer(1:w152) -> (0:w94:i64)
    n45 = To Quad Integer(1:w107) -> (0:w85:i64)
    n46 = To Quad Integer(1:w102) -> (0:w84:i64)
    n47 = To Quad Integer(1:w117) -> (0:w87:i64)
    n48 = To Quad Integer(1:w158) -> (0:w157:i64)
    n49 = To Quad Integer(1:w122) -> (0:w88:i64)
    n50 = To Quad Integer(1:w147) -> (0:w93:i64)
    n51 = To Quad Integer(1:w112) -> (0:w86:i64)
    n52 = To Quad Integer(1:w142) -> (0:w92:i64)
    n53 = To Quad Integer(1:w127) -> (0:w89:i64)
    n54 = To Quad Integer(1:w132) -> (0:w90:i64)
    n55 = To Quad Integer(1:w97) -> (0:w83:i64)
    n56 = for {
      N: w32 -> [_]
      tunnel: w165 -> [w229]
      tunnel: [w228] -> w48 mode=indexing
      tunnel: w157 -> [w227]
      tunnel: [w226] -> w47 mode=indexing
      tunnel: w94 -> [w225]
      tunnel: w93 -> [w223]
      tunnel: w92 -> [w222]
      tunnel: w91 -> [w221]
      tunnel: w90 -> [w220]
      tunnel: w89 -> [w219]
      tunnel: w88 -> [w218]
      tunnel: w87 -> [w217]
      tunnel: w86 -> [w216]
      tunnel: w85 -> [w215]
      tunnel: w84 -> [w214]
      tunnel: w83 -> [w213]
      tunnel: [w212] -> w46 mode=indexing
      tunnel: [w211] -> w45 mode=indexing
      tunnel: [w210] -> w44 mode=indexing
      tunnel: [w209] -> w43 mode=indexing
      tunnel: [w208] -> w42 mode=indexing
      tunnel: [w207] -> w41 mode=indexing
      tunnel: [w206] -> w40 mode=indexing
      tunnel: [w205] -> w39 mode=indexing
      tunnel: [w204] -> w38 mode=indexing
      tunnel: [w203] -> w37 mode=indexing
      tunnel: [w202] -> w36 mode=indexing
      tunnel: [w201] -> w35 mode=indexing
      i -> [w224]
      n57 = Greater?(x=w229, y=w224) -> (0:w228:bool)
      n58 = Greater?(x=w221, y=w224) -> (0:w209:bool)
      n59 = Greater?(x=w225, y=w224) -> (0:w212:bool)
      n60 = Greater?(x=w215, y=w224) -> (0:w203:bool)
      n61 = Greater?(x=w214, y=w224) -> (0:w202:bool)
      n62 = Greater?(x=w217, y=w224) -> (0:w205:bool)
      n63 = Greater?(x=w227, y=w224) -> (0:w226:bool)
      n64 = Greater?(x=w218, y=w224) -> (0:w206:bool)
      n65 = Greater?(x=w223, y=w224) -> (0:w211:bool)
      n66 = Greater?(x=w216, y=w224) -> (0:w204:bool)
      n67 = Greater?(x=w222, y=w224) -> (0:w210:bool)
      n68 = Greater?(x=w219, y=w224) -> (0:w207:bool)
      n69 = Greater?(x=w220, y=w224) -> (0:w208:bool)
      n70 = Greater?(x=w213, y=w224) -> (0:w201:bool)
    }
    n71 = disable-structure shown="Disabled" {
      disable-tunnel: w32 -> [w187 _]
      disable-tunnel: w48 -> [w186 _]
      disable-tunnel: w47 -> [w185 _]
      disable-tunnel: w46 -> [w184 _]
      disable-tunnel: w45 -> [w183 _]
      disable-tunnel: w44 -> [w182 _]
      disable-tunnel: w43 -> [w181 _]
      disable-tunnel: w42 -> [w180 _]
      disable-tunnel: w41 -> [w179 _]
      disable-tunnel: w40 -> [w178 _]
      disable-tunnel: w39 -> [w177 _]
      disable-tunnel: w38 -> [w176 _]
      disable-tunnel: w37 -> [w175 _]
      disable-tunnel: w36 -> [w174 _]
      disable-tunnel: w35 -> [w173 _]
      frame Disabled {
        n72 = for {
          N: w187 -> [_]
          tunnel: w186 -> [_] mode=indexing
          tunnel: w185 -> [w188] mode=indexing
          tunnel: w184 -> [_] mode=indexing
          tunnel: w183 -> [_] mode=indexing
          tunnel: w182 -> [_] mode=indexing
          tunnel: w181 -> [_] mode=indexing
          tunnel: w180 -> [_] mode=indexing
          tunnel: w179 -> [_] mode=indexing
          tunnel: w178 -> [_] mode=indexing
          tunnel: w177 -> [_] mode=indexing
          tunnel: w176 -> [_] mode=indexing
          tunnel: w175 -> [_] mode=indexing
          tunnel: w174 -> [_] mode=indexing
          tunnel: w173 -> [_] mode=indexing
          tunnel: [w190] -> _
          tunnel: [w189] -> _
          n73 = Build Array(w188) -> (w191:bool[])
          n74 = Wait (ms)(milliseconds to wait=u32 10) -> ()  [unwired: 1 out]
          n75 = call-poly <vilib>:"DAQmx Write.vi"("data"=w191) -> ("task out"=w190:refnum<k21>, "error out"=w189:errorcluster)  [unwired: 12 in, 1 out]
        }
      }
      frame Enabled {
      }
    }
    n76 = Bundle(w48, w47, w46, w45, w44, w43, w42, w41, w40, w39, w38, w37, w36, w35) -> (w34:T4)  [unwired: 1 in]
    n77 = Unbundle(w49) -> (w27:bool[], w33:bool[])  [unwired: 12 out]
    n78 = call "Elapsed Time"() -> ("Elapsed Time (s)"=w171:dbl)  [unwired: 12 in, 7 out]
    "Elapsed Time (s)" <- w171
    n79 = for {
      N: w32 -> [_]
      tunnel: w33 -> [w193] mode=indexing
      tunnel: [w196] -> w29
      tunnel: [w195] -> w28
      tunnel: w31 -> [w199]
      tunnel: w30 -> [w198]
      tunnel: w27 -> [w194] mode=indexing
      n80 = Wait (ms)(milliseconds to wait=u32 10) -> ()  [unwired: 1 out]
      n81 = Build Array(w194, w193) -> (w197:bool[])
      n82 = call-poly <vilib>:"DAQmx Write.vi"("task/channels in"=w199, "data"=w197, "error in"=w198) -> ("task out"=w196:refnum<k21>, "error out"=w195:errorcluster)  [unwired: 10 in, 1 out]
      "WinOn 2" <- w193
      "WinOn 1" <- w194
    }
    n83 = Subtract(x=w171, y=w170) -> (x-y=→"Waveform Chart":dbl)
    n84 = Build Array("T5 Setpoint [C]", w64) -> (w145:dbl[])
    n85 = Build Array("T6 Setpoint [C]", w63) -> (w140:dbl[])
    n86 = Build Array("T7 Setpoint [C]", w62) -> (w135:dbl[])
    n87 = Build Array("T8 Setpoint [C]", w61) -> (w130:dbl[])
    n88 = Build Array("T9 Setpoint [C]", w60) -> (w125:dbl[])
    n89 = Build Array("T10 Setpoint [C]", w59) -> (w120:dbl[])
    n90 = Build Array("T11 Setpoint [C]", w58) -> (w115:dbl[])
    n91 = Build Array("T12 Setpoint [C]", w57) -> (w110:dbl[])
    n92 = Build Array("T13 Setpoint [C]", w56) -> (w105:dbl[])
    n93 = Build Array("T14 Setpoint [C]", w55) -> (w100:dbl[])
    n94 = Wait (ms)(milliseconds to wait=u32 1000) -> ()  [unwired: 1 out]
    n95 = Array To Cluster(array=w145) -> (cluster=→"T5":cluster{"[0]":dbl, "[1]":dbl})
    n96 = Array To Cluster(array=w140) -> (cluster=→"T6":cluster{"[0]":dbl, "[1]":dbl})
    n97 = Array To Cluster(array=w135) -> (cluster=→"T7":cluster{"[0]":dbl, "[1]":dbl})
    n98 = Array To Cluster(array=w130) -> (cluster=→"T8":cluster{"[0]":dbl, "[1]":dbl})
    n99 = Array To Cluster(array=w125) -> (cluster=→"T9":cluster{"[0]":dbl, "[1]":dbl})
    n100 = Array To Cluster(array=w120) -> (cluster=→"T10":cluster{"[0]":dbl, "[1]":dbl})
    n101 = Array To Cluster(array=w115) -> (cluster=→"T11":cluster{"[0]":dbl, "[1]":dbl})
    n102 = Array To Cluster(array=w110) -> (cluster=→"T12":cluster{"[0]":dbl, "[1]":dbl})
    n103 = Array To Cluster(array=w105) -> (cluster=→"T13":cluster{"[0]":dbl, "[1]":dbl})
    n104 = Array To Cluster(array=w100) -> (cluster=→"T14":cluster{"[0]":dbl, "[1]":dbl})
  }
  n105 = while {
    stop <- "stop 4" stop-if-true
    n106 = local write "Send Pulse"("Send Pulse 2") -> ()
    n107 = local write "Save File"("Save Loop Data") -> ()
    n108 = Multiply(x="Length of recording (s)", y="Sampling frequency (Hz)") -> (x*y=w359:dbl)
    n109 = call "DAQ Assistant6"("rate"="Sampling frequency (Hz)", "number of samples"=w359) -> ("task out"=w361:refnum<k21>, "data"=w382:dynamicdata)  [unwired: 14 in, 2 out]
    n110 = Split Signals(w382) -> (w370:dynamicdata, w384:dynamicdata, w381:dynamicdata, w367:dynamicdata, w352:dynamicdata, w354:dynamicdata, w353:dynamicdata, w342:dynamicdata)  [unwired: 8 in]
    "Vapor Temp" <- w367
    "Liquid Temp" <- w352
    "Pitot Amps" <- w381
    "Camera Voltage" <- w342
    n111 = case shown="True" "Boolean" {
      tunnel: w361 -> [_ w806]
      tunnel: "Sampling frequency (Hz)" -> [_ w804]
      tunnel: w359 -> [_ w803]
      frame False {
      }
      frame True {
        n112 = call <vilib>:"DAQmx Stop Task.vi"("task/channels in"=w806) -> ("task out"=w805:refnum<k21>)  [unwired: 13 in, 1 out]
        n113 = call-poly <vilib>:"DAQmx Timing.vi"("task/channels in"=w805, "samples per channel"=w803, "rate"=w804) -> ()  [unwired: 11 in, 2 out]
      }
    }
    n114 = xnode "Formula"("V"=w370) -> ("Result"=w376:dynamicdata)  [unwired: 1 in, 1 out]
    n115 = xnode "Set Dynamic Data Attributes"("Signals In"=w370, "Signal Name"="Abs P Volts") -> ("Signals Out"=w369:dynamicdata)  [unwired: 2 in, 1 out]
    n116 = xnode "Formula"("V"=w384) -> ("Result"=w348:dynamicdata)  [unwired: 1 in, 1 out]
    n117 = xnode "Formula"("T"=w367) -> ("Result"=→"Psat vap":dynamicdata)  [unwired: 1 in, 1 out]
    n118 = xnode "Set Dynamic Data Attributes"("Signals In"=w367, "Signal Name"="PG Temp[C]") -> ("Signals Out"=w366:dynamicdata)  [unwired: 2 in, 1 out]
    n119 = xnode "Formula"("I"=w381) -> ("Result"=w343:dynamicdata)  [unwired: 1 in, 1 out]
    n120 = xnode "Formula"("T"=w352) -> ("Result"=→"Psat liq":dynamicdata)  [unwired: 1 in, 1 out]
    n121 = xnode "Formula"("I"=w354) -> ("Result"=→"dP [Pa] W1 to W4":dynamicdata)  [unwired: 1 in, 1 out]
    n122 = xnode "Formula"("I"=w353) -> ("Result"=→"dP [Pa]  W1 to W7":dynamicdata)  [unwired: 1 in, 1 out]
    n123 = xnode "Formula"("T"=w367) -> ("Result"=w385:dynamicdata)  [unwired: 1 in, 1 out]
    n124 = xnode "Formula"("P"=w343) -> ("Result"=w383:dynamicdata)  [unwired: 1 in, 1 out]
    n125 = xnode "Formula"("P"=w343) -> ("Result"=w345:dynamicdata)  [unwired: 1 in, 1 out]
    n126 = xnode "Formula"("dP"=w383, "rho"=w385) -> ("Result"=w379:dynamicdata)  [unwired: 1 in, 1 out]
    "Mass Flow Rate" <- w379
    n127 = Add(x="PG-TS Offset\n[Pa]", y=w348) -> (x+y=w347:dynamicdata)
    "PG to TS dP" <- w347
    "dP to test section" <- w347
    n128 = Add(x="PG Abs Offset", y=w376) -> (x+y=w373:dynamicdata)
    "PG Abs" <- w373
    "Tank Pressure" <- w373
    n129 = Add(x="Pitot Offset [Pa]", y=w345) -> (x+y=w344:dynamicdata)
    "Pitot dP" <- w344
    "dP Pitot Probe" <- w344
    n130 = xnode "Set Dynamic Data Attributes"("Signals In"=w373, "Signal Name"="Adjusted Abs P[Pa]") -> ("Signals Out"=w372:dynamicdata)  [unwired: 2 in, 1 out]
    n131 = xnode "Set Dynamic Data Attributes"("Signals In"=w379, "Signal Name"="m_dot[g/s]") -> ("Signals Out"=w378:dynamicdata)  [unwired: 2 in, 1 out]
    n132 = Merge Signals(w369, w372, w384, w347, w385, w378, w366, w344, w381, w354, w353, w342) -> (w364:dynamicdata)
    n133 = case shown="True" "Save dP data" {
      tunnel: w364 -> [_ w809]
      frame False {
      }
      frame True {
        n134 = call "Write To Measurement File2"("Signals"=w809) -> ("Saving Data"=w807:bool)  [unwired: 16 in, 2 out]
        n135 = Not(x=w807) -> (.not. x?=w808:bool)
        n136 = local write "Save dP data"(w808) -> ()
      }
    }
  }
  n137 = while {
    shift-right: [w1981] -> _
    shift-left: _ -> [w1980]
    stop <- "stop" stop-if-true
    # "Vapor, Liquid Flow Rate\nDev Section Pressure"
    # "Window 3-4 P"
    # "Need to add new pressure sensor on test seciton"
    # "Dev Section P"
    # "liq inlet"
    # "sep tk"
    # "liq tk"
    # "vapor tk"
    # "Calibrations used by Mark for thermocouples:\nIn temp vapor tank:\n(24642*V)+24.36\nIn temp liquid tank:\n(24869*V)+24.24\nIn temp liquid inlet:\n(24775*V)+24.24\nIn temp vapor inlet:\n(24515*V)+24.29"
    n138 = call "Elapsed Time2"() -> ("Elapsed Time (s)"=w1981:dbl)  [unwired: 12 in, 7 out]
    n139 = call "DAQ Assistant3"() -> ("data"=w2153:dynamicdata)  [unwired: 17 in, 2 out]
    n140 = Subtract(x=w1981, y=w1980) -> (x-y=→"Loop Time":dbl)
    n141 = Split Signals(w2153) -> (w2018:dynamicdata, w2076:dynamicdata, w2017:dynamicdata, w2046:dynamicdata, w2150:dynamicdata, w2149:dynamicdata, w2152:dynamicdata, w2151:dynamicdata, w2091:dynamicdata, w2154:dynamicdata, w2155:dynamicdata, w2156:dynamicdata, w2157:dynamicdata, w2158:dynamicdata, w2148:dynamicdata, w2147:dynamicdata, w2142:dynamicdata, w2141:dynamicdata, w2139:dynamicdata, w2090:dynamicdata, w2089:dynamicdata, w2080:dynamicdata, w2079:dynamicdata, w2078:dynamicdata, w2077:dynamicdata, w2016:dynamicdata)  [unwired: 26 in]
    "Numeric" <- w2018
    "Pressure Drop" <- w2139
    n142 = xnode "Output Current to Flow liq"("I"=w2017) -> ("Result"=w2057:dynamicdata)  [unwired: 1 in, 1 out]
    n143 = call "SepLiqInPressure.vi"("Abs. Pressure\nVoltage [V]"=w2152) -> ("Absolute Pressure [kPa]"=w1978:dbl)
    n144 = xnode "Output Current to Flow vapor"("I"=w2018) -> ("Result"=w2065:dynamicdata)  [unwired: 1 in, 1 out]
    n145 = call "GagePressure.vi"("Abs. Pressure\nVoltage [V]"=w2016) -> ("Absolute Pressure [kPa]"=w2015:dbl)  [unwired: 10 in]
    n146 = xnode "Liquid Line Density"("DensCurr"=w2046) -> ("Result"=w2054:dynamicdata)  [unwired: 1 in, 1 out]
    n147 = xnode ("Vapor Line Density")("DensCurr"=w2076) -> ("Result"=w2059:dynamicdata)  [unwired: 1 in, 1 out]
    n148 = call "SepLiqInPressure.vi"("Abs. Pressure\nVoltage [V]"=w2151) -> ("Absolute Pressure [kPa]"=w1987:dbl)
    n149 = call "TemperatureVaporTank.vi"("Temp. Voltage\n[V]"=w2154) -> ("Temp. []"=w2019:dbl)  [unwired: 10 in]
    n150 = call "TemperatureVaporInlet.vi"("Temp. Voltage\n[V]"=w2155) -> ("Temp. []"=w2010:dbl)  [unwired: 10 in]
    n151 = call "TemperatureLiquidTank.vi"("Temp. Voltage\n[V]"=w2156) -> ("Temp. []"=w2039:dbl)  [unwired: 10 in]
    n152 = call "TemperatureVaporTank.vi"("Temp. Voltage\n[V]"=w2158) -> ("Temp. []"=w2037:dbl)  [unwired: 10 in]
    n153 = call "TemperatureVaporTank.vi"("Temp. Voltage\n[V]"=w2147) -> ("Temp. []"=w2005:dbl)  [unwired: 10 in]
    n154 = call "TemperatureVaporTank.vi"("Temp. Voltage\n[V]"=w2090) -> ("Temp. []"=w2027:dbl)  [unwired: 10 in]
    n155 = call "VapTankVapInPressure.vi"("Abs. Pressure\nVoltage [V]"=w2150) -> ("Absolute Pressure [kPa]"=w2023:dbl)
    "Vapor Tank 2\n(need replaced)" <- w2023
    n156 = call "VapTankVapInPressure.vi"("Abs. Pressure\nVoltage [V]"=w2149) -> ("Absolute Pressure [kPa]"=w1983:dbl)
    n157 = call "AbsolutePressure.vi"("Abs. Pressure\nVoltage [V]"=w2148) -> ("Absolute Pressure [kPa]"=w2137:dbl)  [unwired: 10 in]
    "Lower Test Section 2\n(not connected)" <- w2137
    n158 = call "TemperatureVaporTank.vi"("Temp. Voltage\n[V]"=w2142) -> ("Temp. []"=w2138:dbl)  [unwired: 10 in]
    "Vapor Tank Heater Temp. [C]" <- w2138
    n159 = call "TemperatureVaporTank.vi"("Temp. Voltage\n[V]"=w2141) -> ("Temp. []"=w2140:dbl)  [unwired: 10 in]
    "Liquid Tank Heater Temp. [C]" <- w2140
    n160 = call "PressureChange.vi"("Pressure Voltage (V)"=w2139) -> ("Streamwise dP (kPa)"=w2020:dbl)  [unwired: 10 in]
    "Streamwise" <- w2020
    n161 = call "UpperTSPres.vi"("Abs. Pressure\nVoltage [V]"=w2089) -> ("Absolute Pressure [kPa]"=w2074:dbl)  [unwired: 10 in]
    "Upper Test Section 2\n(not connected)" <- w2074
    n162 = call "TemperatureVaporTank.vi"("Temp. Voltage\n[V]"=w2080) -> ("Temp. []"=w2083:dbl)  [unwired: 10 in]
    "Condenser Top" <- w2083
    n163 = call "TemperatureVaporTank.vi"("Temp. Voltage\n[V]"=w2079) -> ("Temp. []"=w2082:dbl)  [unwired: 10 in]
    "Condenser Bottom" <- w2082
    n164 = call "TemperatureVaporTank.vi"("Temp. Voltage\n[V]"=w2078) -> ("Temp. []"=w2081:dbl)  [unwired: 10 in]
    "Evaporator Top" <- w2081
    n165 = call "TemperatureVaporTank.vi"("Temp. Voltage\n[V]"=w2077) -> ("Temp. []"=w2024:dbl)  [unwired: 10 in]
    "Evaporator Bottom" <- w2024
    n166 = xnode "Formula"("P"=w1983) -> ("Result"=w2111:dbl)  [unwired: 1 in, 1 out]
    n167 = To Double Precision Float(number=w2059) -> (double precision float=→"Vapor Line Density [g/cm3]":dbl)
    n168 = To Double Precision Float(number=w2054) -> (double precision float=→"Liquid Line Density [g/cm3]":dbl)
    n169 = call "VapIn.vi"("Abs. Pressure\nVoltage [V]"=w2091) -> ("Absolute Pressure [kPa]"=w2021:dbl)  [unwired: 10 in]
    n170 = xnode "Formula"("P"=w2023) -> ("Result"=w2115:dbl)  [unwired: 1 in, 1 out]
    n171 = xnode "Formula"("P"=w2137) -> ("Result"=w2101:dbl)  [unwired: 1 in, 1 out]
    n172 = xnode "Formula"("P"=w2020) -> ("Result"=w2098:dbl)  [unwired: 1 in, 1 out]
    n173 = xnode "Formula"("P"=w2074) -> ("Result"=w2088:dbl)  [unwired: 1 in, 1 out]
    n174 = call "Statistics2"("Signals"=w2057) -> ("Arithmetic Mean"=w2047:dynamicdata)  [unwired: 25 in, 1 out]
    n175 = call "TemperatureLiquidInlet.vi"("Temp. Voltage\n[V]"=w2157) -> ("Temp. [C]"=w2035:dbl)  [unwired: 10 in]
    n176 = call "Statistics"("Signals"=w2065) -> ("Arithmetic Mean"=w2048:dynamicdata)  [unwired: 25 in, 1 out]
    n177 = Add(x=w1983, y="Liquid Tank P offset") -> (x+y=w2011:dbl)
    "Liquid Tank 2" <- w2011
    n178 = Add(x=w1987, y="Liquid Inlet Offset") -> (x+y=w1985:dbl)
    "Liquid Inlet 2" <- w1985
    n179 = Add(x=w2019, y="Vapor Tank T offset") -> (x+y=w2031:dbl)
    "Vapor Tank" <- w2031
    n180 = Add(x="Liquid Tank T offset", y=w2039) -> (x+y=w2032:dbl)
    "Liquid Tank" <- w2032
    n181 = Add(x=w2037, y="Vapor Inlet T offset") -> (x+y=w2029:dbl)
    "Vapor Inlet" <- w2029
    n182 = Add(x=w2027, y="Upper Test Sec") -> (x+y=w2025:dbl)
    "Upper Test Section" <- w2025
    n183 = Add(x="P atm", y=w2015) -> (x+y=w2013:dbl)
    "Test Section P (Pa)" <- w2013
    n184 = Subtract(x=w2111, y=0.0) -> (x-y=→"Liquid Tank Sat. Temp. [C]":dbl)
    n185 = Add(x=w2010, y="Separator T offset") -> (x+y=w2008:dbl)
    "Separator" <- w2008
    n186 = Add(x=w2021, y="Dev Section P offset") -> (x+y=w2000:dbl)
    "Dev Section" <- w2000
    n187 = Add(x=w2005, y="Lower Test Section offset") -> (x+y=w2007:dbl)
    "Lower Test Section" <- w2007
    n188 = call "Convert from Dynamic Data"("Dynamic Data Type"=w2048, "Channel"=0) -> ("Scalar"=w2003:dbl)  [unwired: 2 in]
    "Vapor Flow Rate [g/s]" <- w2003
    n189 = call "Convert from Dynamic Data2"("Dynamic Data Type"=w2047, "Channel"=0) -> ("Scalar"=w1994:dbl)  [unwired: 2 in]
    "Liquid Flow Rate [g/s]" <- w1994
    n190 = Subtract(x=w2115, y=0.0) -> (x-y=→"Vapor Tank Sat. Temp. [C]":dbl)
    n191 = Subtract(x=w2101, y=0.0) -> (x-y=→"?":dbl)
    n192 = Subtract(x=w2098, y=0.0) -> (x-y=→"?":dbl)
    n193 = Subtract(x=w2088, y=0.0) -> (x-y=→"Upper TS Sat. Temp. [C]":dbl)
    n194 = Add(x=259.15, y=w2035) -> (x+y=w2131:dbl)
    n195 = xnode "Formula"("T_v"=w2008, "P_v"=w2021) -> ("Result"=w2093:dbl)  [unwired: 1 in, 1 out]
    n196 = xnode "Formula"("P"=w1985) -> ("Result"=w2106:dbl)  [unwired: 1 in, 1 out]
    n197 = xnode "Formula"("T"=w2131) -> ("Result"=w2095:dbl)  [unwired: 1 in, 1 out]
    n198 = Add(x="Liquid Inlet T offset", y=w2035) -> (x+y=w2030:dbl)
    "Liquid Inlet" <- w2030
    n199 = Add(x=273.15, y=w2031) -> (x+y=w2116:dbl)
    n200 = Add(x=273.15, y=w2008) -> (x+y=w2122:dbl)
    n201 = Add(x=273.15, y=w2032) -> (x+y=w2124:dbl)
    n202 = Add(x=273.15, y=w2029) -> (x+y=w2118:dbl)
    n203 = Add(x=w2025, y=273.15) -> (x+y=w2084:dbl)
    n204 = xnode "Formula"("m_dot_l"=w1994, "h_l"=w2095, "m_dot_v"=w2003, "h_v"=w2093) -> ("Result"=w2096:dbl)  [unwired: 1 in, 1 out]
    "Mixture Enthalpy" <- w2096
    n205 = case shown="False" "VaporManPID" {
      tunnel: "Vapor Flow Set Point\n[g/s]" -> [w2470 _]
      tunnel: [w2462 w2472] -> w2062
      tunnel: w2003 -> [w2460 _]
      tunnel: "Valve Voltage [V]" -> [w2468 w2472]
      frame False {
        n206 = call <vilib>:"PID Autotuning.vi"("reinitialize? (F)"="reinitialize? (F)", "PID gains"="PID gains", "process variable"=w2460, "setpoint"=w2470) -> ("output"=w2469:dbl)  [unwired: 4 in, 3 out]
        n207 = Cluster To Array(cluster="output range") -> (array=w2466:dbl[])
        n208 = Add(x=w2468, y=w2469) -> (x+y=w2463:dbl)
        n209 = Array Max & Min(array=w2466) -> (max value=w2465:dbl, min value=w2464:dbl)  [unwired: 2 out]
        n210 = In Range and Coerce(upper limit=w2465, x=w2463, lower limit=w2464) -> (coerced(x)=w2462:dbl)  [unwired: 1 out]
      }
      frame True {
      }
    }
    n211 = case shown="True" "LiquidManPID" {
      tunnel: "Liquid Flow Set Point\n[g/s]" -> [w2318 _]
      tunnel: [w2310 w2320] -> w1990
      tunnel: w1994 -> [w2317 _]
      tunnel: "Valve Voltage [V] 2" -> [w2309 w2320]
      frame False {
        n212 = call <vilib>:"PID Autotuning.vi"("reinitialize? (F)"="reinitialize? (F) 2", "PID gains"="PID gains 2", "process variable"=w2317, "setpoint"=w2318) -> ("output"=w2316:dbl)  [unwired: 4 in, 3 out]
        n213 = Cluster To Array(cluster="output range 2") -> (array=w2313:dbl[])
        n214 = Add(x=w2309, y=w2316) -> (x+y=w2315:dbl)
        n215 = Array Max & Min(array=w2313) -> (max value=w2311:dbl, min value=w2312:dbl)  [unwired: 2 out]
        n216 = In Range and Coerce(upper limit=w2311, x=w2315, lower limit=w2312) -> (coerced(x)=w2310:dbl)  [unwired: 1 out]
      }
      frame True {
      }
    }
    n217 = case shown="True" "Boolean 2" {
      tunnel: w2003 -> [w2164 w2167]
      tunnel: w1994 -> [w2165 w2168]
      tunnel: [w2165 w2168] -> w2002
      tunnel: [w2164 w2167] -> w2001
      tunnel: w2000 -> [w2163 w2166]
      tunnel: [w2163 w2166] -> w1999
      frame False {
      }
      frame True {
      }
    }
    n218 = xnode "Formula"("P"=w2000) -> ("Result"=w2028:dbl)  [unwired: 1 in, 1 out]
    n219 = xnode "Formula"("T"=w2116) -> ("Result"=→"Vapor Tank Sat. Pres.":dbl)  [unwired: 1 in, 1 out]
    n220 = xnode "Formula"("T"=w2122) -> ("Result"=→"Vapor Inlet Sat. Pres.":dbl)  [unwired: 1 in, 1 out]
    n221 = xnode "Formula"("T"=w2124) -> ("Result"=→"Liquid Tank Sat. Pres.":dbl)  [unwired: 1 in, 1 out]
    n222 = xnode "Formula"("T"=w2118) -> ("Result"=→"Separator Sat. Pres.":dbl)  [unwired: 1 in, 1 out]
    n223 = xnode "Formula"("T"=w2084) -> ("Result"=w2067:dbl)  [unwired: 1 in, 1 out]
    "Upper TS Sat. Pres." <- w2067
    n224 = Build Array("Vapor Flow Set Point\n[g/s]", w2003) -> (w1997:dbl[])
    n225 = Build Array(w1994, "Liquid Flow Set Point\n[g/s]") -> (w2049:dbl[])
    n226 = Subtract(x=w2106, y=0.0) -> (x-y=→"Liquid Inlet Sat. Temp. [C]":dbl)
    n227 = Add(x=273.15, y=w2008) -> (x+y=w2128:dbl)
    n228 = Add(x=273.15, y=w2007) -> (x+y=w2120:dbl)
    n229 = xnode "Formula"("T"=w2128) -> ("Result"=w2094:dbl)  [unwired: 1 in, 1 out]
    n230 = xnode "Formula"("T"=w2120) -> ("Result"=w2068:dbl)  [unwired: 1 in, 1 out]
    "Lower Test Section Sat. Pres." <- w2068
    n231 = Array To Cluster(array=w1997) -> (cluster=→"Vapor Mass Flow Rate":cluster{"[0]":dbl, "[1]":dbl})
    n232 = Array To Cluster(array=w2049) -> (cluster=→"Liquid Mass Flow Rate":cluster{"[0]":dbl, "[1]":dbl})
    n233 = Subtract(x=w2028, y=0.0) -> (x-y=→"Vapor Inlet Sat. Temp. [C]":dbl)
    n234 = Add(x=273.15, y=w2030) -> (x+y=w2126:dbl)
    n235 = xnode "Formula"("h_mix"=w2096, "h_l"=w2095, "h_v"=w2094) -> ("Result"=→"Quality\n[-]":dbl)  [unwired: 1 in, 1 out]
    n236 = xnode "Formula"("T"=w2126) -> ("Result"=→"Liquid Inlet Sat. Pres.":dbl)  [unwired: 1 in, 1 out]
    n237 = Subtract(x=w2068, y=w2067) -> (x-y=w2073:dbl)
    n238 = Merge Signals(w2002, w2001, w1999) -> (w2004:dynamicdata)
    n239 = Divide(x=w2073, y=2.54) -> (x/y=w2071:dbl)
    n240 = call "Write To Measurement File3"("Signals"=w2004, "Enable"=FALSE) -> ()  [unwired: 15 in, 3 out]
    n241 = Multiply(x=w2071, y=0.678) -> (x*y=→"StaticPressDiff(Pa)":dbl)
    n242 = Boolean To (0,1)(Boolean="VaporOnOff") -> (0, 1=w2063:i16)
    n243 = Boolean To (0,1)(Boolean="LiquidOnOff") -> (0, 1=w2055:i16)
    n244 = To Double Precision Float(number=w2055) -> (double precision float=w1995:dbl)
    n245 = To Double Precision Float(number=w2063) -> (double precision float=w2061:dbl)
    n246 = Multiply(x=w1990, y=w1995) -> (x*y=w1989:dbl)
    "Voltage Out 2" <- w1989
    n247 = xnode "Formula"("V"="Vapor Tank Heater [V]") -> ("Result"=w2159:dbl)  [unwired: 1 in, 1 out]
    n248 = Multiply(x=w2062, y=w2061) -> (x*y=w2060:dbl)
    "Voltage Out" <- w2060
    n249 = call "Simulate Signal4"("Offset"=w1989) -> ("DC"=w2145:dynamicdata)  [unwired: 13 in, 1 out]
    n250 = call "Simulate Signal2"("Offset"=w2159) -> ("DC"=w2143:dynamicdata)  [unwired: 13 in, 1 out]
    "DC" <- w2143
    n251 = xnode "Formula"("V"="Liquid Tank Heater [V]") -> ("Result"=w2160:dbl)  [unwired: 1 in, 1 out]
    n252 = call "Simulate Signal3"("Offset"=w2060) -> ("DC"=w2146:dynamicdata)  [unwired: 13 in, 1 out]
    n253 = call "Simulate Signal"("Offset"=w2160) -> ("DC"=w2144:dynamicdata)  [unwired: 13 in, 1 out]
    n254 = Merge Signals(w2145, w2146, w2143, w2144) -> (w2042:dynamicdata)
    n255 = call "DAQ Assistant"("data"=w2042) -> ()  [unwired: 17 in, 2 out]
    n256 = Add(x=w1978, y="Separator P Offset") -> (x+y=w2022:dbl)
    "Separator 2" <- w2022
    n257 = xnode "Formula"("P"=w2022) -> ("Result"=w1988:dbl)  [unwired: 1 in, 1 out]
    n258 = Merge Signals(w2003, w1994, w2023, w2011, w2022, w1987, w2021, w2020, w2019, w2008, w2039, w2035, w2029, w2137, w2007, w2138, w2140, w2027, w2074, w2083, w2082, w2081, w2024, w2013) -> (w2075:dynamicdata)
    n259 = Subtract(x=w1988, y=0.0) -> (x-y=→"Separator Sat. Temp. [C]":dbl)
    n260 = case shown="True" "Save File" {
      tunnel: w2075 -> [_ w2473]
      frame False {
      }
      frame True {
        n261 = call "Write To Measurement File"("Signals"=w2473) -> ()  [unwired: 16 in, 3 out]
      }
    }
  }
  n262 = while {
    tunnel: [w2963] -> w2
    stop <- "?" stop-if-true
    w2955 = 10178 items=["Continuous Samples"=10123, "Finite Samples"=10178]
    n263 = Build Array("CCW") -> (w2946:bool[])
    n264 = Build Array("Heaters") -> (w2944:bool[])
    n265 = call "Convert to Dynamic Data"("Array"=w2946) -> ("Dynamic Data Type"=w2945:dynamicdata)  [unwired: 3 in]
    n266 = call "Convert to Dynamic Data2"("Array"=w2944) -> ("Dynamic Data Type"=w2943:dynamicdata)  [unwired: 3 in]
    n267 = Merge Signals(w2945, w2943) -> (w2942:dynamicdata)
    n268 = call-poly <vilib>:"DAQmx Create Virtual Channel.vi"("frequency"="Frequency (Hz)", "duty cycle"="Duty Cycle", "counter"="Counter(s)", "idle state"="Idle State", "initial delay"=0.0) -> ("task out"=w2957:refnum<k21>, "error out"=w2956:errorcluster)  [unwired: 9 in]
    n269 = call "Convert from Dynamic Data3"("Dynamic Data Type"=w2942) -> ("Array"=w2941:bool[])  [unwired: 3 in]
    n270 = call "DAQ Assistant4"("data"=w2941) -> ()  [unwired: 17 in, 2 out]
    n271 = call-poly <vilib>:"DAQmx Timing.vi"("task/channels in"=w2957, "sample mode"=w2955, "samples per channel"="Steps", "error in"=w2956) -> ("task out"=w2951:refnum<k21>, "error out"=w2950:errorcluster)  [unwired: 10 in]
    n272 = case shown="True" "Send Pulse" {
      tunnel: [w2964 w2971] -> w2953
      tunnel: [w2965 w2970] -> w2952
      tunnel: w2951 -> [w2965 w2967]
      tunnel: w2950 -> [w2964 w2966]
      frame False {
      }
      frame True {
        n273 = call <vilib>:"DAQmx Start Task.vi"("task/channels in"=w2967, "error in"=w2966) -> ("task out"=w2969:refnum<k21>, "error out"=w2968:errorcluster)  [unwired: 12 in]
        n274 = while {
          tunnel: w2969 -> [w2979]
          tunnel: w2968 -> [w2978]
          tunnel: [w2975] -> w2970
          tunnel: [w2974] -> w2971
          i -> [w2973]
          stop <- w2976 stop-if-true
          n275 = call <vilib>:"DAQmx Is Task Done.vi"("task/channels in"=w2979, "error in"=w2978) -> ("task out"=w2975:refnum<k21>, "error out"=w2974:errorcluster)  [unwired: 11 in, 1 out]
          n276 = Unbundle By Name(w2974) -> ("status"=w2977:bool)
          n277 = Or(x=w2977, y="?") -> (x .or. y?=w2976:bool)
          "Loop iterations" <- w2973
        }
      }
    }
    n278 = call <vilib>:"DAQmx Clear Task.vi"("task in"=w2952, "error in"=w2953) -> ("error out"=w2963:errorcluster)  [unwired: 13 in]
  }
  n279 = property class="TabCtl (strict)"("BG Color"=u32 9868950 ("Color"), "FG Color"=u32 13816530 ("Color")) -> ()  [unwired: 2 in, 2 out]
  n280 = call <vilib>:"Simple Error Handler.vi"("type of dialog (OK msg:1)"=w1, "error in (no error)"=w2) -> ()  [unwired: 3 in, 5 out]
  n281 = call <vilib>:"DAQmx Stop Task.vi"("task/channels in"=w16, "error in"=w15) -> ("task out"=w22:refnum<k21>, "error out"=w21:errorcluster)  [unwired: 12 in]
  n282 = call <vilib>:"DAQmx Clear Task.vi"("task in"=w22, "error in"=w21) -> ("error out"=→"error out":errorcluster)  [unwired: 13 in]
  n283 = call-poly <vilib>:"DAQmx Write.vi"("task/channels in"=w6, "data"=bool[] [FALSE], "error in"=w5) -> ("task out"=w8:refnum<k21>, "error out"=w7:errorcluster)  [unwired: 10 in, 1 out]
  n284 = call <vilib>:"DAQmx Stop Task.vi"("task/channels in"=w8, "error in"=w7) -> ("task out"=w14:refnum<k21>, "error out"=w13:errorcluster)  [unwired: 12 in]
  n285 = call <vilib>:"DAQmx Clear Task.vi"("task in"=w14, "error in"=w13) -> ("error out"=→"error out 2":errorcluster)  [unwired: 13 in]
